vi "New Items_Collect.vi"(0 "With Parent Tag?":bool, 4 "Name":string[](array[string]), 6 "Item Indent":i32, 7 "Items In":T1[](array[typedef]), 8 "Child Item Text":cluster{"2-D String":string[]}[](array[cluster]), 9 "Symbols":i32[](array[numeric]), 10 "Parent Tag":string, 11 "Tag":string[](array[string])) -> (5 "Items Out":T1[](array[typedef]))   [LabVIEW 2024]
doc: "This VI Collecting the Items \nFot \"Add to Multiple Items To End\"\nAlso Combined the Parent Tag and\nTag to become Child Tag"
uses:
  Ancestor Class/Front Panel Container/Tree/Tree/Type Def/Tree Item.ctl
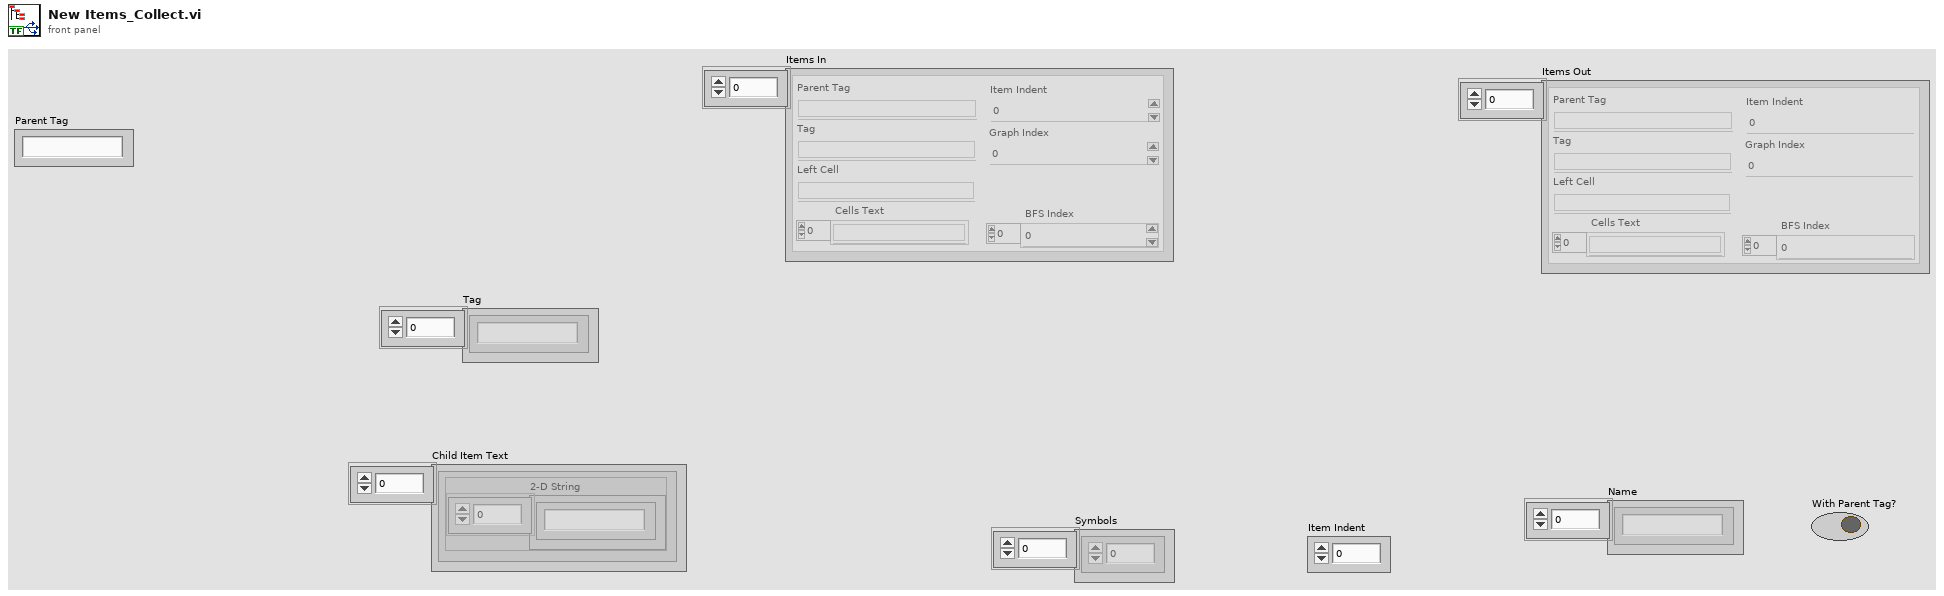
[diagram p1: front panel]
types:
  T1 = typedef "Tree Item.ctl" = cluster{"Parent Tag":string, "Tag":string, "Left Cell":string, "Cells Text":string[], "BFS Index":i32[], "Graph Index":i32, "Item Indent":i32}
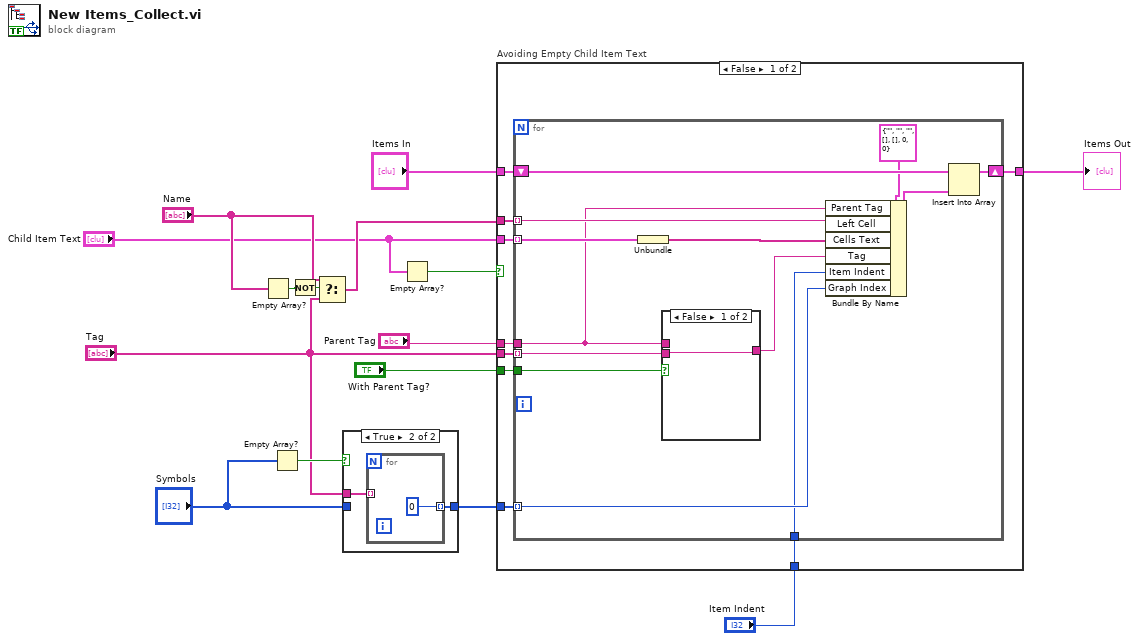
[diagram p0: block diagram]
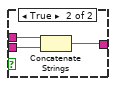
[diagram p2: hidden frame]
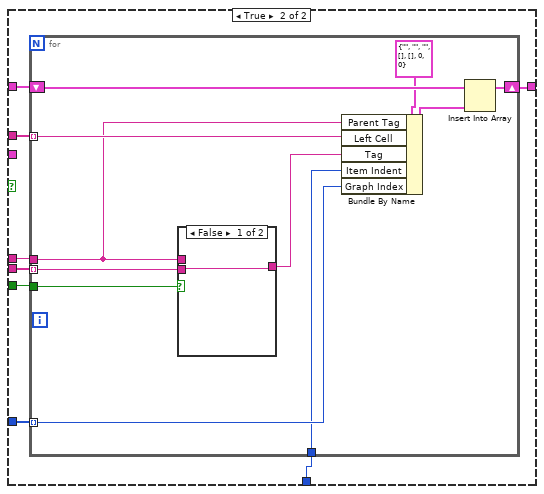
[diagram p3: hidden frame]
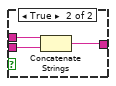
[diagram p4: hidden frame]
diagram:
  n1 = Empty Array?(array="Name") -> (empty?=w10:bool)
  n2 = Empty Array?(array="Symbols") -> (empty?=w8:bool)
  n3 = Not(x=w10) -> (.not. x?=w11:bool)
  n4 = Select(t="Name", s=w11, f="Tag") -> (s? t:f=w12:string[])
  n5 = case shown="True" w8 {
    tunnel: "Symbols" -> [w16 _]
    tunnel: [w16 w17] -> w6
    tunnel: "Tag" -> [_ w18]
    frame False {
    }
    frame True {
      n6 = for {
        tunnel: w18 -> [_] mode=indexing
        tunnel: [0] -> w17 mode=indexing
      }
    }
  }
  n7 = Empty Array?(array="Child Item Text") -> (empty?=w2:bool)
  n8 = case "Avoiding Empty Child Item Text" shown="False" w2 {
    tunnel: "Parent Tag" -> [w28 w50]
    tunnel: "Items In" -> [w27 w53]
    tunnel: [w26 w52] -> w13
    tunnel: w12 -> [w25 w51]
    tunnel: w6 -> [w24 w47]
    tunnel: "Tag" -> [w23 w49]
    tunnel: "Child Item Text" -> [w22 _]
    tunnel: "With Parent Tag?" -> [w21 w48]
    tunnel: "Item Indent" -> [w20 w46]
    frame False {
      n9 = for {
        tunnel: w28 -> [w29]
        tunnel: w23 -> [w41] mode=indexing
        tunnel: w22 -> [w35] mode=indexing
        shift-right: [w37] -> w26
        shift-left: w27 -> [w39]
        tunnel: w24 -> [w36] mode=indexing
        tunnel: w25 -> [w32] mode=indexing
        tunnel: w21 -> [w31]
        tunnel: w20 -> [w30]
        n10 = Unbundle(w35) -> ("2-D String"=w34:string[])
        n11 = case shown="False" w31 {
          tunnel: w29 -> [_ w45]
          tunnel: w41 -> [w42 w44]
          tunnel: [w42 w43] -> w40
          frame False {
          }
          frame True {
            n12 = Concatenate Strings(w45, w44) -> (w43:string)
          }
        }
        n13 = Bundle By Name(cluster=T1 {"Parent Tag"="", "Tag"="", "Left Cell"="", "Cells Text"=[], "BFS Index"=[], "Graph Index"=0, "Item Indent"=0} ("TreeItem"), "Parent Tag"=w29, "Left Cell"=w32, "Cells Text"=w34, "Tag"=w40, "Item Indent"=w30, "Graph Index"=w36) -> (w38:T1)
        n14 = Insert Into Array(array=w39, new element=w38) -> (w37:T1[])  [unwired: 1 in]
      }
    }
    frame True {
      n15 = for {
        tunnel: w50 -> [w54]
        tunnel: w49 -> [w64] mode=indexing
        shift-right: [w60] -> w52
        shift-left: w53 -> [w62]
        tunnel: w47 -> [w59] mode=indexing
        tunnel: w51 -> [w57] mode=indexing
        tunnel: w48 -> [w56]
        tunnel: w46 -> [w55]
        n16 = case shown="False" w56 {
          tunnel: w54 -> [_ w68]
          tunnel: w64 -> [w65 w67]
          tunnel: [w65 w66] -> w63
          frame False {
          }
          frame True {
            n17 = Concatenate Strings(w68, w67) -> (w66:string)
          }
        }
        n18 = Bundle By Name(cluster=T1 {"Parent Tag"="", "Tag"="", "Left Cell"="", "Cells Text"=[], "BFS Index"=[], "Graph Index"=0, "Item Indent"=0} ("TreeItem"), "Parent Tag"=w54, "Left Cell"=w57, "Tag"=w63, "Item Indent"=w55, "Graph Index"=w59) -> (w61:T1)
        n19 = Insert Into Array(array=w62, new element=w61) -> (w60:T1[])  [unwired: 1 in]
      }
    }
  }
  "Items Out" <- w13
